vi "Aim test.vi"(0 "List box Aiming":string[](array[string]), 1 "Check path or camera":bool, 2 "Exposure":dbl, 5 "error in 3":errorcluster, 6 "Image":T1(plugin-control), 7 "Camera Refnum in":T3) -> (14 "Aiming Result":T2, 15 "Image 2":T1(plugin-control), 16 "Camera Refnum in 2":T3, 19 "error out 3":errorcluster)   [LabVIEW 2020]
uses:
  <vilib>/userdefined/High Color/IMAQdx.ctl
  <vilib>/vision/NI_Vision_Development_Module.lvlib
  <vilib>/vision/driver/NI_Vision_Acquisition_Software.lvlib
  <resource>/objmgr/imaqdx.rc
  General/Daq code/S-IO Channel List.ctl
panel:
  out "Elaphsed time":dbl
  out "millisecond timer value":u32
  out "Aiminjg name":string
  out "Y axis distance to move :":dbl
  out "X axis distance to move :":dbl
  out "RESULT":bool caption="Result"
  out "Y direction":bool
  out "X direction":bool
  out "Y":i64
  out "X":i64
  out "Y":i64
  out "X":i64
  in  "Boolean":bool
  out "Buffer Number":u32
  out "Frame Rate":dbl(knob) scale=0.0..100.0
  in  "Transperancy":dbl(slide) scale=0.0..1.0
  out "new picture":picture
  in  "stop":bool
  out "Cross Hair Coordinates 2":cluster{"X":i32, "Y":i32}
  out "Image Out 4":T1(plugin-control)
  out "Particle Measurements (Pixels) 4":dbl[][](array[numeric]) format="%.2f"
  out "Particle Measurements (Pixels) 3":dbl[][](array[numeric]) format="%.2f"
  out "Cross Hair Coordinates":cluster{"X":i32, "Y":i32}
  out "Particle Measurements (Pixels) 2":dbl[][](array[numeric]) format="%.2f"
  out "Particle Measurements (Pixels)":dbl[][](array[numeric]) format="%.2f"
  out "error out 2":errorcluster
  out "Image Out 3":T1(plugin-control)
  # "Status"
  # "Expected Value"
  # "Actual Value"
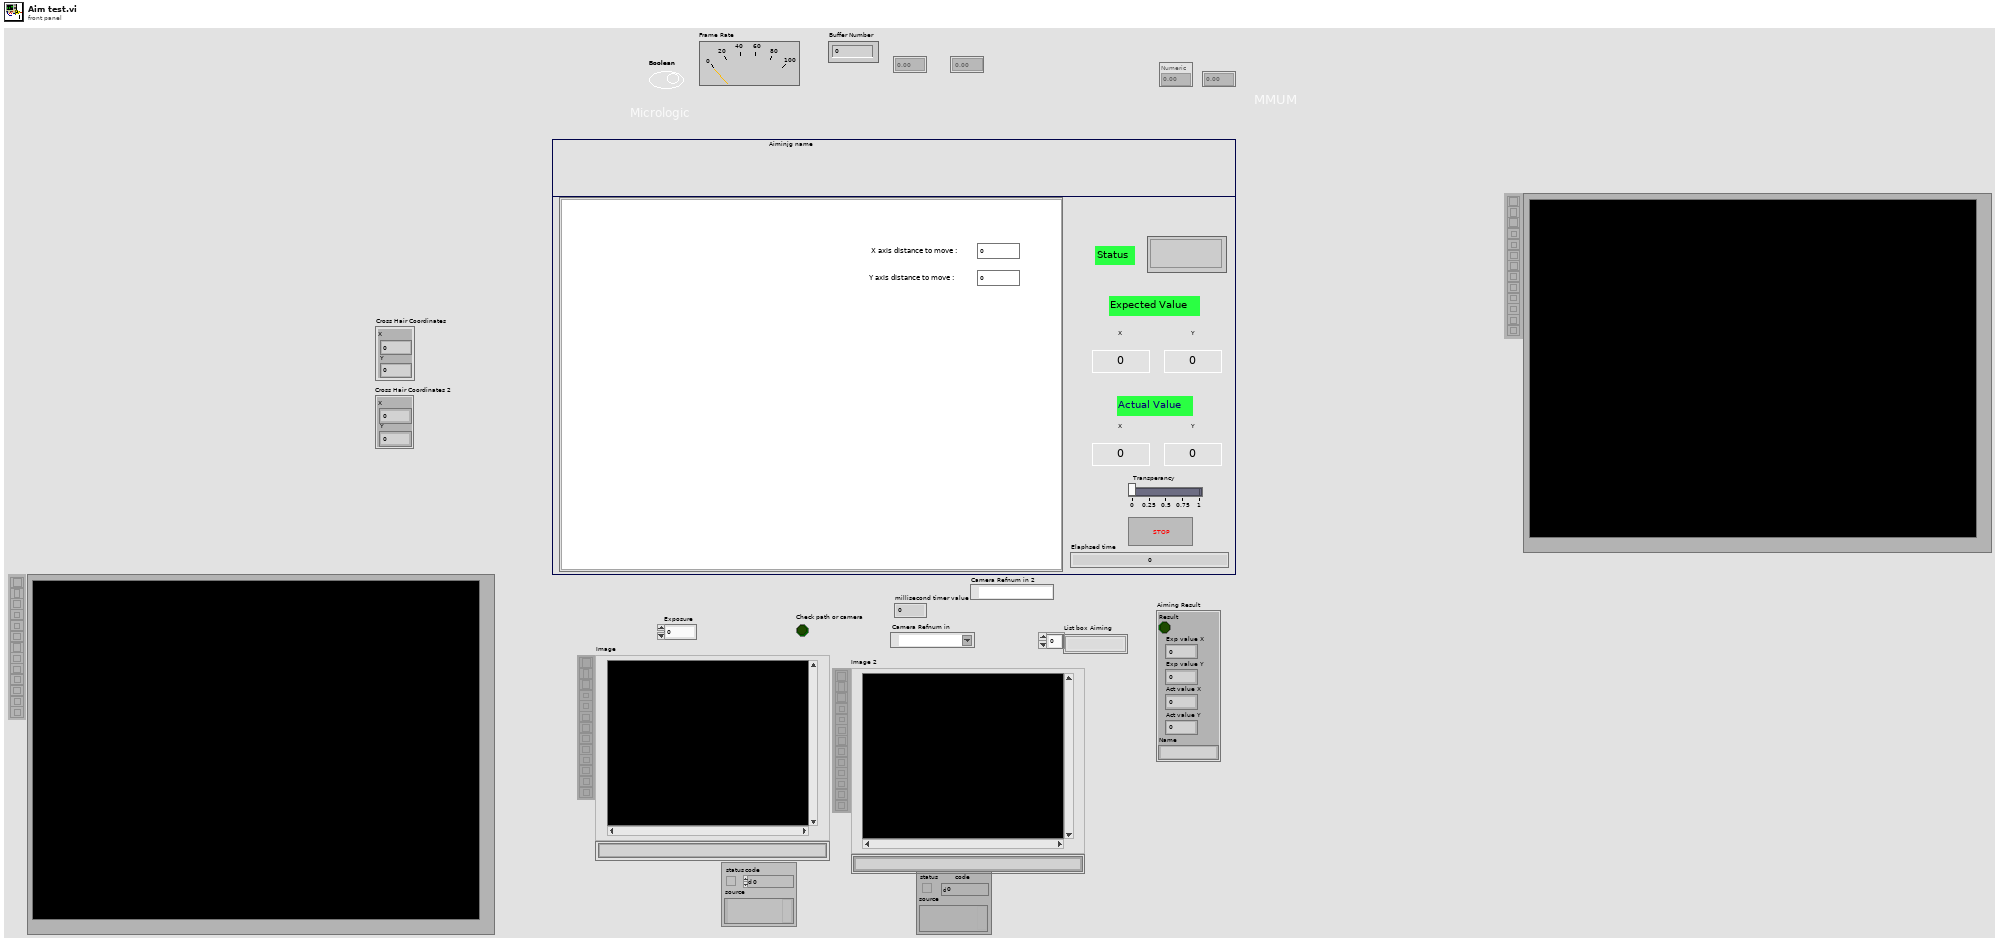
[diagram p1: front panel]
types:
  T1 = typedef "IMAQ Image.ctl" = refnum<image>
  T2 = cluster{"Result":bool, "Exp value X":i64, "Exp value Y":i64, "Act value X ":i64, "Act value Y ":i64, "Name":string}
  T3 = typedef "IMAQdx.ctl" = refnum<k21>
  T4 = typedef "Image Type" = u32
  T5 = typedef "Particle Parameters" = i32
  T6 = typedef "S-IO Channel List.ctl" = enum16{"Initialsation", "Reset All DOs", "Reset all expet lamp", "Read DI", "Read DI - line name", "Write DO", "Write DO - Line name", "Read DO", "Close"}
  T7 = cluster{"Left":i32, "Top":i32, "Right":i32, "Bottom":i32}
  T8 = typedef "imagedata.ctl" = cluster{"image type":i32, "image depth":i32, "image":u8[], "mask":u8[], "colors":u32[], "Rectangle":cluster{"left":i16, "top":i16, "right":i16, "bottom":i16}}
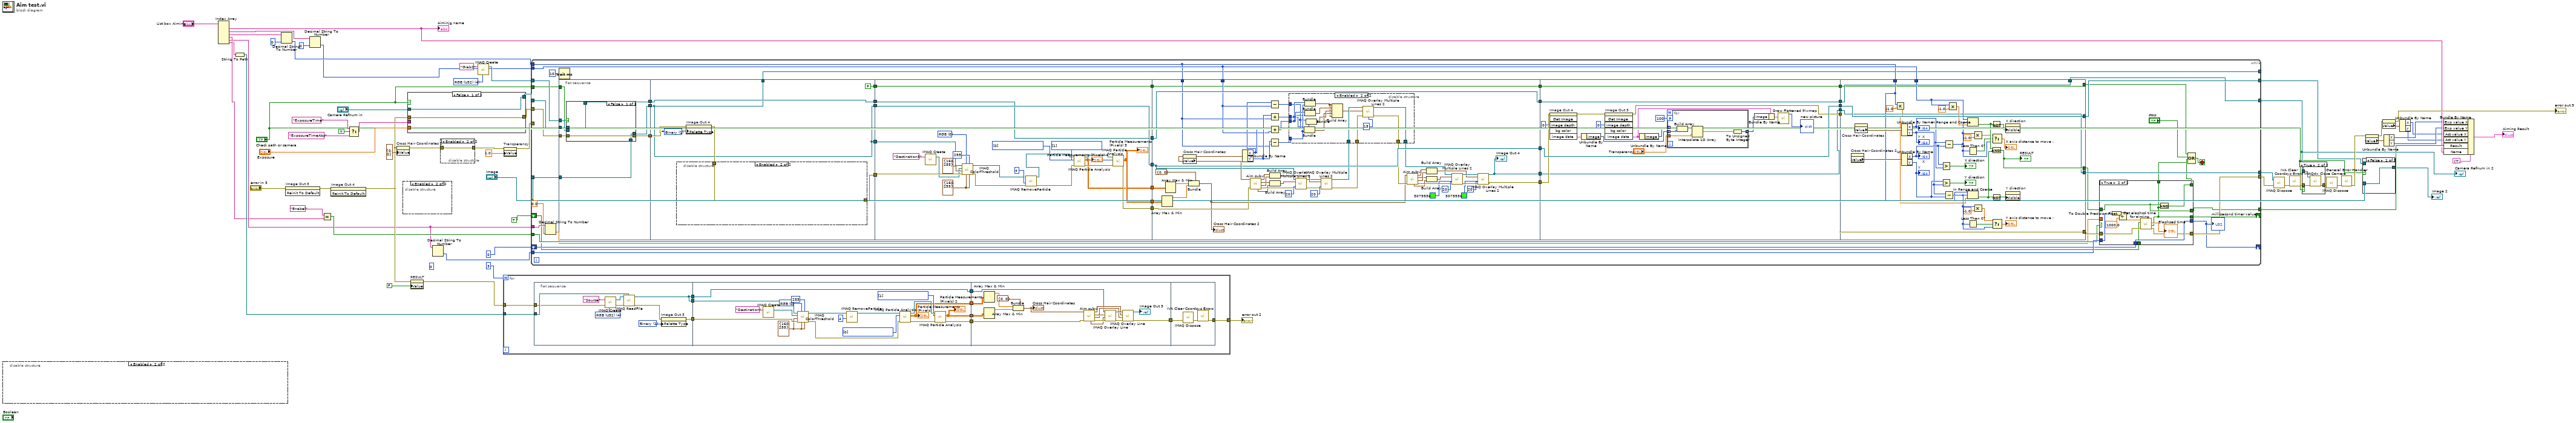
[diagram p0: block diagram]
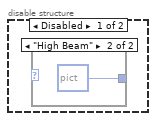
[diagram p3: hidden frame]
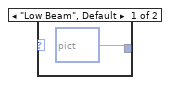
[diagram p4: hidden frame]
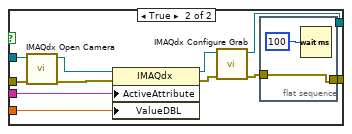
[diagram p6: hidden frame]
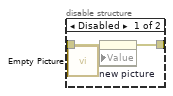
[diagram p7: hidden frame]
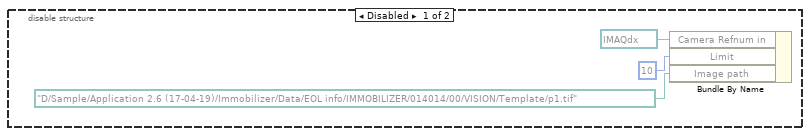
[diagram p8: hidden frame]
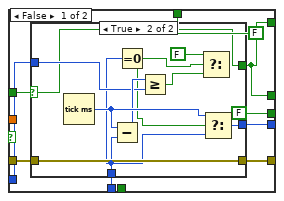
[diagram p9: hidden frame]
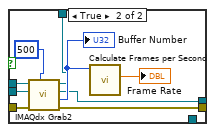
[diagram p11: hidden frame]
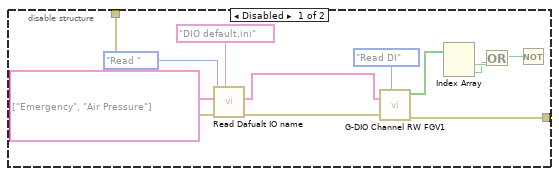
[diagram p12: hidden frame]
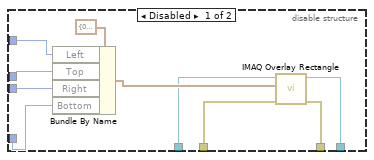
[diagram p13: hidden frame]
diagram:
  (unwired) i64 0 ("time out")
  w44 = T4 4 items=["Grayscale (U8)", "Grayscale (I16)", "Grayscale (SGL)", "Complex (CSG)", "RGB (U32)", "HSL (U32)", "RGB (U64)", "Grayscale (U16)"] ("Image Type")
  n1 = disable-structure shown="Enabled" {
    frame Disabled {
      n2 = Bundle By Name("Camera Refnum in"=T3 "cam1", "Limit"=i64 10, "Image path"=path "D:/Sample/Application 2.6 (17-04-19)/Immobilizer/Data/EOL info/IMMOBILIZER/014014/00/VISION/Template/p1.tif") -> ()  [unwired: 1 in, 1 out]
    }
    frame Enabled {
    }
  }
  n3 = Index Array(array="List box Aiming") -> (element #1=w20:string, element #2=w26:string, element #3=w27:string, element #4=w2:string, element #5=w3:string, element #6=w1:string)  [unwired: 6 in]
  "Aiminjg name" <- w20
  n4 = String To Path(string=w1) -> (path=w22:path)
  n5 = Decimal String To Number(string=w27, default (0L)=i64 0 ("Limit B")) -> (number=w25:i64)  [unwired: 1 in, 1 out]
  n6 = invoke on="Image Out 3" class="ImageControl" method="Reinit To Default"(error in="error in 3") -> (error out=w32:errorcluster)  [unwired: 2 in, 2 out]
  n7 = Decimal String To Number(string=w26, default (0L)=i64 0 ("Limit B")) -> (number=w24:i64)  [unwired: 1 in, 1 out]
  n8 = Equal?(x="Enabel" ("element"), y=w2) -> (x = y?=w4:bool)
  n9 = invoke on="Image Out 4" class="ImageControl" method="Reinit To Default"(error in=w32) -> (error out=w31:errorcluster)  [unwired: 2 in, 2 out]
  n10 = Select(t="ExposureTime" ("ActiveAttribute"), s=TRUE, f="ExposureTimeAbs" ("ActiveAttribute")) -> (s? t:f=w37:string)
  n11 = property on="Cross Hair Coordinates 2" class="Clust (strict)"(error in=w31, "Value"=cluster{"X":i32, "Y":i32} {"X"=0, "Y"=0} ("Cross Hair Coordinates 2")) -> (error out=w47:errorcluster)  [unwired: 1 in, 1 out]
  n12 = disable-structure shown="Enabled" {
    frame Disabled {
      n13 = case shown="\"High Beam\"" {
        selector: _ -> [_ _]
        tunnel: [picture bytes[1461630] ("new picture") picture bytes[1461630] ("new picture")] -> _
        frame "Low Beam", Default {
        }
        frame "High Beam" {
        }
      }
    }
    frame Enabled {
    }
  }
  n14 = case shown="False" "Check path or camera" {
    tunnel: [w70 w81] -> w63
    tunnel: "Camera Refnum in" -> [w70 w76]
    tunnel: [w69 w74] -> w43
    tunnel: w37 -> [_ w73]
    tunnel: w31 -> [w69 w72]
    tunnel: "Exposure" -> [_ w71]
    frame False {
    }
    frame True {
      n15 = call <vilib>:"IMAQdx Open Camera.vi"("error in"=w72, "Session In"=w76) -> ("error out"=w79:errorcluster, "Session Out"=w80:T3)  [unwired: 1 in, 7 out]
      n16 = property class="IMAQdx"(reference=w80, error in=w79, "ActiveAttribute"=w73, "ValueDBL"=w71) -> (reference out=w78:T3, error out=w77:errorcluster)
      n17 = call <vilib>:"IMAQdx Configure Grab.vi"("error in"=w77, "Session In"=w78) -> ("error out"=w75:errorcluster, "Session Out"=w81:T3)  [unwired: 1 in, 7 out]
      n18 = flat-sequence {
        tunnel: [w83] -> w74
        tunnel: w75 -> [w83]
        frame #0 {
          n19 = Wait (ms)(milliseconds to wait=u32 100) -> ()  [unwired: 1 out]
        }
      }
    }
  }
  n20 = property on="RESULT" class="Bool (strict)"(error in=w31, "Value"=FALSE ("RESULT")) -> (error out=w53:errorcluster)  [unwired: 1 in, 1 out]
  n21 = Decimal String To Number(string=w3) -> (number=w6:i32)  [unwired: 2 in, 1 out]
  n22 = disable-structure shown="Enabled" {
    disable-tunnel: w47 -> [w86 w87]
    disable-tunnel: [w85 w87] -> w46
    frame Disabled {
      n23 = call "Empty Picture"() -> ("empty picture"=w84:picture)
      n24 = property on="new picture" class="Pict"(error in=w86, "Value"=w84) -> (error out=w85:errorcluster)  [unwired: 1 in, 1 out]
    }
    frame Enabled {
    }
  }
  n25 = call "IMAQ Create"("Image Name"="Grab2", "Image Type"=w44) -> ("New Image"=w51:T1)  [unwired: 2 in, 2 out]
  n26 = for {
    N: 3 -> [_]
    tunnel: w22 -> [w90]
    tunnel: [w89] -> w49
    tunnel: w53 -> [w88]
    n27 = flat-sequence {
      tunnel: [w101] -> w98
      tunnel: [w103] -> w97
      tunnel: [w101] -> w96
      tunnel: w90 -> [w100]
      tunnel: w88 -> [w99]
      tunnel: w98 -> [w109]
      tunnel: w97 -> [w126]
      tunnel: [w119] -> w95
      tunnel: [w118] -> w94
      tunnel: [w117] -> w93
      tunnel: [w116] -> w92
      tunnel: w96 -> [w116]
      tunnel: w95 -> [w142]
      tunnel: [w130] -> w91
      tunnel: w94 -> [w134]
      tunnel: w93 -> [w133]
      tunnel: w92 -> [w132]
      tunnel: w91 -> [w147]
      tunnel: [w145] -> w89
      frame #0 {
        w105 = u32 1 items=["Grayscale", "Binary", "Gradient", "Rainbow", "Temperature", "User Defined", "Binary 16 Bit", "Gradient 16 Bit", "Rainbow 16 Bit", "Temperature 16 Bit", "User Defined 16 Bit"] ("Palette Type")
        w106 = T4 4 items=["Grayscale (U8)", "Grayscale (I16)", "Grayscale (SGL)", "Complex (CSG)", "RGB (U32)", "HSL (U32)", "RGB (U64)", "Grayscale (U16)"] ("Image Type")
        n28 = call "IMAQ Create"("Image Name"="Source", "Image Type"=w106, "error in (no error)"=w99) -> ("New Image"=w108:T1, "error out"=w107:errorcluster)  [unwired: 1 in, 1 out]
        n29 = call "IMAQ ReadFile"("File Path"=w100, "error in (no error)"=w107, "Image"=w108) -> ("error out"=w104:errorcluster, "Image Out"=w101:T1)  [unwired: 2 in, 5 out]
        n30 = property on="Image Out 3" class="ImageControl"(error in=w104, "Palette:Palette Type"=w105) -> (error out=w103:errorcluster)  [unwired: 1 in, 1 out]
      }
      frame #1 {
        w111 = u16 0 items=["RGB", "HSL", "HSV", "HSI"] ("Color Mode")
        w121 = T5[] [1] items=["Center of Mass X", "Center of Mass Y", "First Pixel X", "First Pixel Y", "Bounding Rect Left", "Bounding Rect Top", "Bounding Rect Right", "Bounding Rect Bottom", "Max Feret Diameter Start X", "Max Feret Diameter Start Y", "Max Feret Diameter End X", "Max Feret Diameter End Y", "Max Horiz. Segment Length Left", "Max Horiz. Segment Length Right", "Max Horiz. Segment Length Row", "-", "Bounding Rect Width", "Bounding Rect Height", "Bounding Rect Diagonal", "Perimeter", "Convex Hull Perimeter", "Holes' Perimeter", "Max Feret Diameter", "Equivalent Ellipse Major Axis", "Equivalent Ellipse Minor Axis", "Equivalent Ellipse Minor Axis (Feret)", "Equivalent Rect Long Side", "Equivalent Rect Short Side", "Equivalent Rect Diagonal", "Equivalent Rect Short Side (Feret)", "Average Horiz. Segment Length", "Average Vert. Segment Length", "Hydraulic Radius", "Waddel Disk Diameter", "-", "Area", "Holes' Area", "Particle & Holes' Area", "Convex Hull Area", "Image Area", "-", "Number of Holes", "Number of Horiz. Segments", "Number of Vert. Segments", "-", "Orientation", "Max Feret Diameter Orientation", "-", "% Area/Image Area", "% Area/(Particle & Holes' Area)", "Ratio of Equivalent Ellipse Axes", "Ratio of Equivalent Rect Sides", "-", "Elongation Factor", "Compactness Factor", "Heywood Circularity Factor", "Type Factor", "-", "Sum X", "Sum Y", "Sum XX", "Sum XY", "Sum YY", "Sum XXX", "Sum XXY", "Sum XYY", "Sum YYY", "-", "Moment of Inertia XX", "Moment of Inertia XY", "Moment of Inertia YY", "Moment of Inertia XXX", "Moment of Inertia XXY", "Moment of Inertia XYY", "Moment of Inertia YYY", "Norm. Moment of Inertia XX", "Norm. Moment of Inertia XY", "Norm. Moment of Inertia YY", "Norm. Moment of Inertia XXX", "Norm. Moment of Inertia XXY", "Norm. Moment of Inertia XYY", "Norm. Moment of Inertia YYY", "Hu Moment 1", "Hu Moment 2", "Hu Moment 3", "Hu Moment 4", "Hu Moment 5", "Hu Moment 6", "Hu Moment 7"] ("Pixel Measurements")
        w113 = cluster{"Lower value":i32, "Upper value":i32} {"Lower value"=160, "Upper value"=255} ("Red or Hue Range")
        w127 = T5[] [0] items=["Center of Mass X", "Center of Mass Y", "First Pixel X", "First Pixel Y", "Bounding Rect Left", "Bounding Rect Top", "Bounding Rect Right", "Bounding Rect Bottom", "Max Feret Diameter Start X", "Max Feret Diameter Start Y", "Max Feret Diameter End X", "Max Feret Diameter End Y", "Max Horiz. Segment Length Left", "Max Horiz. Segment Length Right", "Max Horiz. Segment Length Row", "-", "Bounding Rect Width", "Bounding Rect Height", "Bounding Rect Diagonal", "Perimeter", "Convex Hull Perimeter", "Holes' Perimeter", "Max Feret Diameter", "Equivalent Ellipse Major Axis", "Equivalent Ellipse Minor Axis", "Equivalent Ellipse Minor Axis (Feret)", "Equivalent Rect Long Side", "Equivalent Rect Short Side", "Equivalent Rect Diagonal", "Equivalent Rect Short Side (Feret)", "Average Horiz. Segment Length", "Average Vert. Segment Length", "Hydraulic Radius", "Waddel Disk Diameter", "-", "Area", "Holes' Area", "Particle & Holes' Area", "Convex Hull Area", "Image Area", "-", "Number of Holes", "Number of Horiz. Segments", "Number of Vert. Segments", "-", "Orientation", "Max Feret Diameter Orientation", "-", "% Area/Image Area", "% Area/(Particle & Holes' Area)", "Ratio of Equivalent Ellipse Axes", "Ratio of Equivalent Rect Sides", "-", "Elongation Factor", "Compactness Factor", "Heywood Circularity Factor", "Type Factor", "-", "Sum X", "Sum Y", "Sum XX", "Sum XY", "Sum YY", "Sum XXX", "Sum XXY", "Sum XYY", "Sum YYY", "-", "Moment of Inertia XX", "Moment of Inertia XY", "Moment of Inertia YY", "Moment of Inertia XXX", "Moment of Inertia XXY", "Moment of Inertia XYY", "Moment of Inertia YYY", "Norm. Moment of Inertia XX", "Norm. Moment of Inertia XY", "Norm. Moment of Inertia YY", "Norm. Moment of Inertia XXX", "Norm. Moment of Inertia XXY", "Norm. Moment of Inertia XYY", "Norm. Moment of Inertia YYY", "Hu Moment 1", "Hu Moment 2", "Hu Moment 3", "Hu Moment 4", "Hu Moment 5", "Hu Moment 6", "Hu Moment 7"] ("Pixel Measurements")
        n31 = call "IMAQ Create"("Image Name"="Destination") -> ("New Image"=w123:T1)  [unwired: 3 in, 2 out]
        n32 = call "IMAQ ColorThreshold"("Blue or Luma or Val or Inten Range"=w113, "Replace Value"=255, "Green or Sat Range"=w113, "Color Mode"=w111, "error in (no error)"=w126, "Red or Hue Range"=w113, "Image Dst"=w123, "Image Src"=w109) -> ("error out"=w125:errorcluster, "Image Dst Out"=w110:T1)  [unwired: 2 in]
        n33 = call "IMAQ RemoveParticle"("Number of Erosion"=4, "Image Src"=w110) -> ("Image Dst Out"=w115:T1)  [unwired: 5 in, 4 out]
        n34 = call "IMAQ Particle Analysis"("error in (no error)"=w125, "Pixel Measurements"=w127, "Image"=w115) -> ("error out"=w120:errorcluster, "Particle Measurements (Pixels)"=w118:dbl[][], "Image Out (duplicate)"=w122:T1)  [unwired: 3 in, 3 out]
        "Particle Measurements (Pixels)" <- w118
        n35 = call "IMAQ Particle Analysis"("error in (no error)"=w120, "Pixel Measurements"=w121, "Image"=w122) -> ("error out"=w119:errorcluster, "Particle Measurements (Pixels)"=w117:dbl[][])  [unwired: 3 in, 4 out]
        "Particle Measurements (Pixels) 2" <- w117
      }
      frame #2 {
        n36 = Array Max & Min(array=w134) -> (max value=w144:dbl)  [unwired: 3 out]
        n37 = Array Max & Min(array=w133) -> (max value=w143:dbl)  [unwired: 3 out]
        n38 = Bundle(cluster=cluster{"X":i32, "Y":i32} {"X"=0, "Y"=0} ("Cross Hair Coordinates 2"), "X"=w144, "Y"=w143) -> (w128:cluster{"X":i32, "Y":i32})
        "Cross Hair Coordinates" <- w128
        n39 = call "Aim subvi.vi"("Coordinates"=w128, "error in (no error)"=w142) -> ("Cluster 3"=w135:cluster{"X":i32, "Y":i32}, "Cluster 2"=w138:cluster{"X":i32, "Y":i32}, "Cluster 4"=w137:cluster{"X":i32, "Y":i32}, "Cluster"=w136:cluster{"X":i32, "Y":i32}, "error out"=w141:errorcluster)  [unwired: 4 in]
        n40 = call "IMAQ Overlay Line"("error in (no error)"=w141, "End Point"=w135, "Start Point"=w137, "Image"=w132) -> ("error out"=w140:errorcluster, "Image Out"=w139:T1)  [unwired: 6 in]
        n41 = call "IMAQ Overlay Line"("error in (no error)"=w140, "End Point"=w136, "Start Point"=w138, "Image"=w139) -> ("error out"=w130:errorcluster, "Image Out"=→"Image Out 3":T1)  [unwired: 6 in]
      }
      frame #3 {
        n42 = call "IMAQ Dispose"("error in (no error)"=w147) -> ("error out"=w146:errorcluster)  [unwired: 2 in, 3 out]
        n43 = call <vilib>:"IVA Clear Coordsys Errors.vi"("error in (no error)"=w146) -> ("error out"=w145:errorcluster)  [unwired: 10 in]
      }
    }
  }
  "error out 2" <- w49
  n44 = property on="Transperancy" class="Slide (strict)"(error in=w46, "Value"=1.0 ("Transperancy")) -> (error out=w57:errorcluster)  [unwired: 1 in, 1 out]
  n45 = while {
    tunnel: w43 -> [w191]
    tunnel: [w170] -> w59
    tunnel: w24 -> [w172]
    tunnel: w57 -> [_]
    tunnel: [w173] -> w50
    tunnel: w25 -> [w171]
    shift-right: [w168] -> _
    shift-left: u32 0 ("millisecond timer value") -> [w161]
    tunnel: w6 -> [w167]
    tunnel: w63 -> [w190]
    tunnel: [w178] -> w41
    tunnel: w51 -> [w177]
    tunnel: [w185] -> w10
    tunnel: w3 -> [w160]
    tunnel: w4 -> [w158]
    shift-right: [w157] -> _
    shift-left: TRUE ("Elaphshed time") -> [w156]
    tunnel: [w152] -> w35
    tunnel: "Check path or camera" -> [w150]
    tunnel: "Image" -> [w149]
    tunnel: [w148] -> _
    stop <- w180 stop-if-true
    n46 = Decimal String To Number(string=w160, default (0L)=0.0) -> (number=w155:dbl)  [unwired: 1 in, 1 out]
    n47 = flat-sequence {
      tunnel: [w239] -> w193
      tunnel: [w238] -> w192
      tunnel: w191 -> [w243]
      tunnel: w190 -> [w242]
      tunnel: [w241] -> w186
      tunnel: w177 -> [w240]
      tunnel: w150 -> [w237]
      tunnel: w149 -> [w236]
      tunnel: [w256] -> w201
      tunnel: [w259] -> w200
      tunnel: [w256] -> w199
      tunnel: w193 -> [w256]
      tunnel: w192 -> [w262]
      tunnel: [w261] -> w187
      tunnel: w186 -> [w261]
      tunnel: [FALSE] -> w163
      tunnel: [w256] -> w148
      tunnel: w201 -> [w276]
      tunnel: w200 -> [w285]
      tunnel: [w293] -> w198
      tunnel: [w288] -> w197
      tunnel: [w289] -> w196
      tunnel: [w292] -> w195
      tunnel: w199 -> [w292]
      tunnel: [w287] -> w188
      tunnel: w187 -> [w287]
      tunnel: [w280] -> w164
      tunnel: w163 -> [w280]
      tunnel: w198 -> [w331]
      tunnel: w197 -> [w345]
      tunnel: w196 -> [w344]
      tunnel: w195 -> [w332]
      tunnel: [w343] -> w189
      tunnel: w188 -> [w343]
      tunnel: [w332] -> w184
      tunnel: [w305] -> w176
      tunnel: [w307] -> w175
      tunnel: w172 -> [w333]
      tunnel: w171 -> [w301]
      tunnel: [w299] -> w165
      tunnel: w164 -> [w299]
      tunnel: w189 -> [w378]
      tunnel: w184 -> [w377]
      tunnel: [w378] -> w183
      tunnel: [w377] -> w182
      tunnel: [w376] -> w181
      tunnel: w176 -> [w375]
      tunnel: w175 -> [w374]
      tunnel: [w374] -> w174
      tunnel: [w373] -> w166
      tunnel: w165 -> [w373]
      tunnel: [w427] -> w169
      tunnel: [w428] -> w185
      tunnel: [w429] -> w178
      tunnel: w183 -> [w429]
      tunnel: w182 -> [w428]
      tunnel: w181 -> [w427]
      tunnel: w172 -> [w402]
      tunnel: [w401] -> w153
      tunnel: w174 -> [w400]
      tunnel: [w400] -> w173
      tunnel: w171 -> [w398]
      tunnel: [w396] -> w162
      tunnel: w166 -> [w396]
      frame #0 {
        n48 = case shown="False" w237 {
          tunnel: w243 -> [w245 w253]
          tunnel: w242 -> [w246 w252]
          tunnel: [w246 w251] -> w241
          tunnel: w240 -> [_ w250]
          tunnel: [w244 w248] -> w239
          tunnel: [w245 w247] -> w238
          tunnel: w236 -> [w244 _]
          frame False {
          }
          frame True {
            n49 = call <vilib>:"IMAQdx Grab2.vi"("Timeout (ms)"=500, "error in"=w253, "Image In"=w250, "Session In"=w252) -> ("error out"=w247:errorcluster, "Buffer Number Out"=w254:u32, "Image Out"=w248:T1, "Session Out"=w251:T3)  [unwired: 4 in]
            "Buffer Number" <- w254
            n50 = call <vilib>:"Calculate Frames per Second.vi"("Buffer Number"=w254) -> ("Processed Frames/s"=→"Frame Rate":dbl)  [unwired: 8 in, 2 out]
          }
        }
      }
      frame #1 {
        w257 = u32 1 items=["Grayscale", "Binary", "Gradient", "Rainbow", "Temperature", "User Defined", "Binary 16 Bit", "Gradient 16 Bit", "Rainbow 16 Bit", "Temperature 16 Bit", "User Defined 16 Bit"] ("Palette Type")
        n51 = property on="Image Out 4" class="ImageControl"(error in=w262, "Palette:Palette Type"=w257) -> (error out=w260:errorcluster)  [unwired: 1 in, 1 out]
        n52 = disable-structure shown="Enabled" {
          disable-tunnel: w260 -> [w270 w275]
          disable-tunnel: [w269 w275] -> w259
          frame Disabled {
            n53 = call "Read Dafualt IO name.vi"("Default Control"="DIO default.ini", "error in (no error)"=w270, "Input/output name"=string[] ["Emergency", "Air Pressure"], "Read/ Write"=enum16{"INI", "Read ", "Write"}."Read ") -> ("error out"=w263:errorcluster, "Value"=w274:string[])  [unwired: 6 in]
            n54 = call "G-DIO Channel RW FGV1.vi"("Command"=S-IO_Channel_List."Read DI", "error in (no error)"=w263, "DIO Names"=w274) -> ("error out"=w269:errorcluster, "Write status"=w267:bool[])  [unwired: 6 in, 1 out]
            n55 = Index Array(array=w267) -> (element #1=w266:bool, element #2=w265:bool)  [unwired: 2 in]
            n56 = Or(x=w266, y=w265) -> (x .or. y?=w264:bool)
            n57 = Not(x=w264) -> ()  [unwired: 1 out]
          }
          frame Enabled {
          }
        }
      }
      frame #2 {
        w279 = u16 0 items=["RGB", "HSL", "HSV", "HSI"] ("Color Mode")
        w295 = T5[] [1] items=["Center of Mass X", "Center of Mass Y", "First Pixel X", "First Pixel Y", "Bounding Rect Left", "Bounding Rect Top", "Bounding Rect Right", "Bounding Rect Bottom", "Max Feret Diameter Start X", "Max Feret Diameter Start Y", "Max Feret Diameter End X", "Max Feret Diameter End Y", "Max Horiz. Segment Length Left", "Max Horiz. Segment Length Right", "Max Horiz. Segment Length Row", "-", "Bounding Rect Width", "Bounding Rect Height", "Bounding Rect Diagonal", "Perimeter", "Convex Hull Perimeter", "Holes' Perimeter", "Max Feret Diameter", "Equivalent Ellipse Major Axis", "Equivalent Ellipse Minor Axis", "Equivalent Ellipse Minor Axis (Feret)", "Equivalent Rect Long Side", "Equivalent Rect Short Side", "Equivalent Rect Diagonal", "Equivalent Rect Short Side (Feret)", "Average Horiz. Segment Length", "Average Vert. Segment Length", "Hydraulic Radius", "Waddel Disk Diameter", "-", "Area", "Holes' Area", "Particle & Holes' Area", "Convex Hull Area", "Image Area", "-", "Number of Holes", "Number of Horiz. Segments", "Number of Vert. Segments", "-", "Orientation", "Max Feret Diameter Orientation", "-", "% Area/Image Area", "% Area/(Particle & Holes' Area)", "Ratio of Equivalent Ellipse Axes", "Ratio of Equivalent Rect Sides", "-", "Elongation Factor", "Compactness Factor", "Heywood Circularity Factor", "Type Factor", "-", "Sum X", "Sum Y", "Sum XX", "Sum XY", "Sum YY", "Sum XXX", "Sum XXY", "Sum XYY", "Sum YYY", "-", "Moment of Inertia XX", "Moment of Inertia XY", "Moment of Inertia YY", "Moment of Inertia XXX", "Moment of Inertia XXY", "Moment of Inertia XYY", "Moment of Inertia YYY", "Norm. Moment of Inertia XX", "Norm. Moment of Inertia XY", "Norm. Moment of Inertia YY", "Norm. Moment of Inertia XXX", "Norm. Moment of Inertia XXY", "Norm. Moment of Inertia XYY", "Norm. Moment of Inertia YYY", "Hu Moment 1", "Hu Moment 2", "Hu Moment 3", "Hu Moment 4", "Hu Moment 5", "Hu Moment 6", "Hu Moment 7"] ("Pixel Measurements")
        w282 = cluster{"Lower value":i32, "Upper value":i32} {"Lower value"=160, "Upper value"=255} ("Red or Hue Range")
        w298 = T5[] [0] items=["Center of Mass X", "Center of Mass Y", "First Pixel X", "First Pixel Y", "Bounding Rect Left", "Bounding Rect Top", "Bounding Rect Right", "Bounding Rect Bottom", "Max Feret Diameter Start X", "Max Feret Diameter Start Y", "Max Feret Diameter End X", "Max Feret Diameter End Y", "Max Horiz. Segment Length Left", "Max Horiz. Segment Length Right", "Max Horiz. Segment Length Row", "-", "Bounding Rect Width", "Bounding Rect Height", "Bounding Rect Diagonal", "Perimeter", "Convex Hull Perimeter", "Holes' Perimeter", "Max Feret Diameter", "Equivalent Ellipse Major Axis", "Equivalent Ellipse Minor Axis", "Equivalent Ellipse Minor Axis (Feret)", "Equivalent Rect Long Side", "Equivalent Rect Short Side", "Equivalent Rect Diagonal", "Equivalent Rect Short Side (Feret)", "Average Horiz. Segment Length", "Average Vert. Segment Length", "Hydraulic Radius", "Waddel Disk Diameter", "-", "Area", "Holes' Area", "Particle & Holes' Area", "Convex Hull Area", "Image Area", "-", "Number of Holes", "Number of Horiz. Segments", "Number of Vert. Segments", "-", "Orientation", "Max Feret Diameter Orientation", "-", "% Area/Image Area", "% Area/(Particle & Holes' Area)", "Ratio of Equivalent Ellipse Axes", "Ratio of Equivalent Rect Sides", "-", "Elongation Factor", "Compactness Factor", "Heywood Circularity Factor", "Type Factor", "-", "Sum X", "Sum Y", "Sum XX", "Sum XY", "Sum YY", "Sum XXX", "Sum XXY", "Sum XYY", "Sum YYY", "-", "Moment of Inertia XX", "Moment of Inertia XY", "Moment of Inertia YY", "Moment of Inertia XXX", "Moment of Inertia XXY", "Moment of Inertia XYY", "Moment of Inertia YYY", "Norm. Moment of Inertia XX", "Norm. Moment of Inertia XY", "Norm. Moment of Inertia YY", "Norm. Moment of Inertia XXX", "Norm. Moment of Inertia XXY", "Norm. Moment of Inertia XYY", "Norm. Moment of Inertia YYY", "Hu Moment 1", "Hu Moment 2", "Hu Moment 3", "Hu Moment 4", "Hu Moment 5", "Hu Moment 6", "Hu Moment 7"] ("Pixel Measurements")
        n58 = call "IMAQ Create"("Image Name"="Destination5") -> ("New Image"=w278:T1)  [unwired: 3 in, 2 out]
        n59 = call "IMAQ ColorThreshold"("Blue or Luma or Val or Inten Range"=w282, "Replace Value"=255, "Green or Sat Range"=w282, "Color Mode"=w279, "error in (no error)"=w285, "Red or Hue Range"=cluster{"Lower value":i32, "Upper value":i32} {"Lower value"=160, "Upper value"=255}, "Image Dst"=w278, "Image Src"=w276) -> ("error out"=w284:errorcluster, "Image Dst Out"=w277:T1)  [unwired: 2 in]
        n60 = call "IMAQ RemoveParticle"("error in (no error)"=w284, "Number of Erosion"=4, "Image Src"=w277) -> ("error out"=w286:errorcluster, "Image Dst Out"=w291:T1)  [unwired: 4 in, 3 out]
        n61 = call "IMAQ Particle Analysis"("error in (no error)"=w286, "Pixel Measurements"=w298, "Image"=w291) -> ("error out"=w294:errorcluster, "Particle Measurements (Pixels)"=w288:dbl[][], "Image Out (duplicate)"=w296:T1)  [unwired: 3 in, 3 out]
        "Particle Measurements (Pixels) 4" <- w288
        n62 = call "IMAQ Particle Analysis"("error in (no error)"=w294, "Pixel Measurements"=w295, "Image"=w296) -> ("error out"=w293:errorcluster, "Particle Measurements (Pixels)"=w289:dbl[][])  [unwired: 3 in, 4 out]
        "Particle Measurements (Pixels) 3" <- w289
      }
      frame #3 {
        n63 = Array Max & Min(array=w344) -> (max value=w346:dbl)  [unwired: 3 out]
        n64 = Array Max & Min(array=w345) -> (max value=w347:dbl)  [unwired: 3 out]
        n65 = property on="Cross Hair Coordinates" class="Clust (strict)"() -> ("Value"=w334:cluster{"X":i32, "Y":i32})  [unwired: 2 in, 2 out]
        n66 = Bundle(cluster=cluster{"X":i32, "Y":i32} {"X"=0, "Y"=0} ("Cross Hair Coordinates 2"), "X"=w347, "Y"=w346) -> (w300:cluster{"X":i32, "Y":i32})
        "Cross Hair Coordinates 2" <- w300
        n67 = Unbundle By Name(w334) -> ("X"=w339:i32, "Y"=w338:i32)
        n68 = call "Aim subvi.vi"("Coordinates"=w334, "error in (no error)"=w331) -> ("Cluster 3"=w329:cluster{"X":i32, "Y":i32}, "Cluster 2"=w322:cluster{"X":i32, "Y":i32}, "Cluster 4"=w330:cluster{"X":i32, "Y":i32}, "Cluster"=w321:cluster{"X":i32, "Y":i32}, "error out"=w335:errorcluster)  [unwired: 4 in]
        n69 = Subtract(x=w339, y=w333) -> (x-y=w340:i64)
        n70 = Add(x=w338, y=w301) -> (x+y=w337:i64)
        n71 = Add(x=w339, y=w333) -> (x+y=w341:i64)
        n72 = Subtract(x=w338, y=w301) -> (x-y=w336:i64)
        n73 = Build Array(w322, w321) -> (w325:cluster{"X":i32, "Y":i32}[])
        n74 = Build Array(w330, w329) -> (w328:cluster{"X":i32, "Y":i32}[])
        n75 = call "IMAQ Overlay Multiple Lines 2"("Image"=w332, "Line End Points"=w328, "error in (no error)"=w335, "Width"=u32 20) -> ("Image Out"=w320:T1, "error out"=w319:errorcluster)  [unwired: 10 in]
        n76 = call "IMAQ Overlay Multiple Lines 2"("Image"=w320, "Line End Points"=w325, "error in (no error)"=w319, "Width"=u32 20) -> ("Image Out"=w324:T1, "error out"=w323:errorcluster)  [unwired: 10 in]
        n77 = disable-structure shown="Enabled" {
          disable-tunnel: w341 -> [w355 w367]
          disable-tunnel: w340 -> [w354 w366]
          disable-tunnel: w337 -> [w353 w358]
          disable-tunnel: w336 -> [w352 w365]
          disable-tunnel: w324 -> [w351 w369]
          disable-tunnel: w323 -> [w350 w368]
          disable-tunnel: [w349 w371] -> w308
          disable-tunnel: [w348 w370] -> w306
          frame Disabled {
            n78 = Bundle By Name(cluster=T7 {"Left"=0, "Top"=0, "Right"=0, "Bottom"=0} ("Rectangle"), "Left"=w354, "Top"=w353, "Right"=w355, "Bottom"=w352) -> (w356:T7)
            n79 = call "IMAQ Overlay Rectangle"("error in (no error)"=w350, "Rectangle"=w356, "Image"=w351) -> ("error out"=w348:errorcluster, "Image Out"=w349:T1)  [unwired: 7 in]
          }
          frame Enabled {
            n80 = Bundle(w366, w365) -> (w362:cluster{i64, i64})  [unwired: 1 in]
            n81 = Bundle(w367, w365) -> (w361:cluster{i64, i64})  [unwired: 1 in]
            n82 = Bundle(w367, w358) -> (w364:cluster{i64, i64})  [unwired: 1 in]
            n83 = Bundle(w366, w358) -> (w363:cluster{i64, i64})  [unwired: 1 in]
            n84 = Build Array(w361, w364, w363, w362, w361) -> (w360:cluster{i64, i64}[])
            n85 = call "IMAQ Overlay Multiple Lines 2"("Image"=w369, "Line End Points"=w360, "error in (no error)"=w368, "Width"=u32 15) -> ("Image Out"=w371:T1, "error out"=w370:errorcluster)  [unwired: 10 in]
          }
        }
        n86 = call "Aim subvi.vi"("Coordinates"=w300, "error in (no error)"=w306) -> ("Cluster 3"=w302:cluster{"X":i32, "Y":i32}, "Cluster 2"=w315:cluster{"X":i32, "Y":i32}, "Cluster 4"=w310:cluster{"X":i32, "Y":i32}, "Cluster"=w316:cluster{"X":i32, "Y":i32}, "error out"=w309:errorcluster)  [unwired: 4 in]
        n87 = Build Array(w315, w316) -> (w314:cluster{"X":i32, "Y":i32}[])
        n88 = Build Array(w310, w302) -> (w311:cluster{"X":i32, "Y":i32}[])
        n89 = call "IMAQ Overlay Multiple Lines 2"("Image"=w308, "Line End Points"=w311, "Color"=u32 3079936, "error in (no error)"=w309, "Width"=u32 20) -> ("Image Out"=w317:T1, "error out"=w318:errorcluster)  [unwired: 9 in]
        n90 = call "IMAQ Overlay Multiple Lines 2"("Image"=w317, "Line End Points"=w314, "Color"=u32 3079936, "error in (no error)"=w318, "Width"=u32 20) -> ("Image Out"=w307:T1, "error out"=w305:errorcluster)  [unwired: 9 in]
        "Image Out 4" <- w307
      }
      frame #4 {
        n91 = invoke on="Image Out 4" class="ImageControl" method="Get Image"(error in=w375, "image depth"=0 ("Image Depth")) -> (error out=w389:errorcluster, "image data"=w388:T8)  [unwired: 4 in, 4 out]
        n92 = Unbundle By Name(w388) -> ("image"=w384:u8[])
        n93 = invoke on="Image Out 3" class="ImageControl" method="Get Image"(error in=w389, "image depth"=0 ("Image Depth")) -> (error out=w376:errorcluster, "image data"=w387:T8)  [unwired: 4 in, 4 out]
        n94 = Unbundle By Name(w387) -> ("image"=w383:u8[])
        n95 = for {
          tunnel: w384 -> [w395] mode=indexing
          tunnel: w383 -> [w394] mode=indexing
          tunnel: [w391] -> w382 mode=indexing
          tunnel: "Transperancy" -> [w390]
          workers-P: 100 -> [_]
          n96 = Build Array(w394, w395) -> (w393:u8[])
          n97 = Interpolate 1D Array(1:w390, 2:w393) -> (0:w392:dbl)
          n98 = To Unsigned Byte Integer(number=w392) -> (unsigned 8bit integer=w391:u8)
        }
        n99 = Bundle By Name(cluster=w387, "image"=w382) -> (w386:T8)
        n100 = call <vilib>:"Draw Flattened Pixmap.vi"("image data"=w386) -> ("new picture"=→"new picture":picture)  [unwired: 1 in, 7 out]
      }
      frame #5 {
        n101 = property on="Cross Hair Coordinates 2" class="Clust (strict)"() -> ("Value"=w403:cluster{"X":i32, "Y":i32})  [unwired: 2 in, 2 out]
        n102 = property on="Cross Hair Coordinates" class="Clust (strict)"() -> ("Value"=w407:cluster{"X":i32, "Y":i32})  [unwired: 2 in, 2 out]
        n103 = Multiply(x=w398, y=-1.0 ("upper limit")) -> (x*y=w397:dbl)
        n104 = Unbundle By Name(w407) -> ("X"=w409:i32, "Y"=w411:i32)
        "X" <- w409
        "Y" <- w411
        n105 = Unbundle By Name(w403) -> ("X"=w414:i32, "Y"=w413:i32)
        "Y" <- w413
        "X" <- w414
        n106 = Greater?(x=w414, y=w409) -> (0:→"X direction":bool)
        n107 = Greater?(x=w413, y=w411) -> (0:→"Y direction":bool)
        n108 = Subtract(x=w409, y=w414) -> (x-y=w422:i32)
        n109 = Subtract(x=w411, y=w413) -> (x-y=w420:i32)
        n110 = Multiply(x=w402, y=-1.0 ("upper limit")) -> (x*y=w408:dbl)
        n111 = In Range and Coerce(upper limit=w402, x=w422, lower limit=w408) -> (In Range?=w423:bool)  [unwired: 1 out]
        n112 = In Range and Coerce(upper limit=w398, x=w420, lower limit=w397) -> (In Range?=w424:bool)  [unwired: 1 out]
        n113 = Less Than 0?(x=w422) -> (x < 0?=w415:bool)
        n114 = Less Than 0?(x=w420) -> (x < 0?=w419:bool)
        n115 = Multiply(x=w422, y=-1.0 ("upper limit")) -> (x*y=w417:dbl)
        n116 = Multiply(x=w420, y=-1.0 ("upper limit")) -> (x*y=w418:dbl)
        n117 = Not(x=w423) -> (.not. x?=w425:bool)
        n118 = And(x=w423, y=w424) -> (x .and. y?=w401:bool)
        "RESULT" <- w401
        n119 = Not(x=w424) -> (.not. x?=w426:bool)
        n120 = Select(t=w417, s=w415, f=w422) -> (s? t:f=→"X axis distance to move :":dbl)
        n121 = Select(t=w418, s=w419, f=w420) -> (s? t:f=→"Y axis distance to move :":dbl)
        n122 = property on="X direction" class="Bool"("Visible"=w425) -> ()  [unwired: 2 in, 2 out]
        n123 = property on="Y direction" class="Bool"("Visible"=w426) -> ()  [unwired: 2 in, 2 out]
      }
    }
    n124 = Wait (ms)(milliseconds to wait=u32 10) -> ()  [unwired: 1 out]
    n125 = case shown="True" w158 {
      tunnel: [w210 w233] -> w170
      tunnel: w169 -> [w209 w234]
      tunnel: [w208 w235] -> w168
      tunnel: w167 -> [w207 w229]
      tunnel: w153 -> [w206 w230]
      tunnel: w161 -> [w205 w235]
      tunnel: [w203 w231] -> w154
      tunnel: [FALSE ("Elaphshed time") w226] -> w157
      tunnel: w156 -> [_ w232]
      tunnel: w155 -> [_ _]
      tunnel: [w203 w230] -> w152
      tunnel: [FALSE ("Elaphshed time") w226] -> w151
      frame False {
        n126 = case shown="True" w206 {
          selector: w206 -> [w212 w214]
          tunnel: [w213 w223] -> w210
          tunnel: w209 -> [w213 w223]
          tunnel: [w212 w214] -> w203
          tunnel: [w211 w220] -> w208
          tunnel: w205 -> [w211 w216]
          tunnel: w207 -> [_ w217]
          frame False {
          }
          frame True {
            n127 = Tick Count (ms)() -> (millisecond timer value=w222:u32)
            n128 = Subtract(x=w222, y=w216) -> (x-y=w221:u32)
            n129 = Equal To 0?(x=w216) -> (x = 0?=w215:bool)
            n130 = Greater Or Equal?(x=w221, y=w217) -> (x >= y?=w219:bool)
            n131 = Select(t=FALSE, s=w215, f=w219) -> ()  [unwired: 1 out]
            n132 = Select(t=w222, s=w215, f=w216) -> (s? t:f=w220:u32)
          }
        }
      }
      frame True {
        n133 = To Double Precision Float(number=w229) -> (double precision float=w228:dbl)
        n134 = Divide(x=w228, y=1000.0) -> (x/y=w225:dbl)
        n135 = call "Get elaphsd time for aiming.vi"("Error in"=w234, "Reset"=w232, "Target time"=w225) -> ("Errorout"=w233:errorcluster, "Elaphshed time"=w226:bool, "Elaphsed time"=→"Elaphsed time":dbl)  [unwired: 6 in]
        n136 = And(x=w230, y=w226) -> (x .and. y?=w231:bool)
      }
    }
    "millisecond timer value" <- w168
    n137 = Compound Arithmetic op=OR(w162, "stop", w154, w151) -> (w180:bool)
  }
  "Camera Refnum in 2" <- w41
  n138 = call "IMAQ Dispose"("Image"=w50, "error in (no error)"=w59) -> ("error out"=w61:errorcluster)  [unwired: 1 in, 3 out]
  n139 = call <vilib>:"IVA Clear Coordsys Errors.vi"("error in (no error)"=w61) -> ("error out"=w60:errorcluster)  [unwired: 10 in]
  n140 = case shown="True" "Check path or camera" {
    tunnel: w60 -> [w430 w433]
    tunnel: [w430 w432] -> w42
    tunnel: w41 -> [_ w431]
    frame False {
    }
    frame True {
      n141 = call <vilib>:"IMAQdx Close Camera.vi"("error in"=w433, "Session In"=w431) -> ("error out"=w432:errorcluster)  [unwired: 9 out]
    }
  }
  n142 = call "IMAQ Dispose"("error in (no error)"=w42) -> ("error out"=w62:errorcluster)  [unwired: 5 in]
  n143 = call <vilib>:"General Error Handler.vi"("error in (no error)"=w62) -> ("error out"=w55:errorcluster)  [unwired: 2 in, 12 out]
  n144 = case shown="False" "Check path or camera" {
    tunnel: w10 -> [_ w435]
    tunnel: [w434 w435] -> w9
    tunnel: "Image" -> [w434 _]
    frame False {
    }
    frame True {
    }
  }
  "Image 2" <- w9
  n145 = property on="Cross Hair Coordinates" class="Clust (strict)"(error in=w55) -> (error out=w19:errorcluster, "Value"=w18:cluster{"X":i32, "Y":i32})  [unwired: 1 in, 1 out]
  n146 = property on="Cross Hair Coordinates 2" class="Clust (strict)"(error in=w19) -> (error out=→"error out 3":errorcluster, "Value"=w15:cluster{"X":i32, "Y":i32})  [unwired: 1 in, 1 out]
  n147 = Unbundle By Name(w18) -> ("X"=w17:i32, "Y"=w16:i32)
  n148 = Unbundle By Name(w15) -> ("X"=w14:i32, "Y"=w13:i32)
  n149 = Bundle By Name(cluster=T2 {"Result"=TRUE, "Exp value X"=0, "Exp value Y"=0, "Act value X "=0, "Act value Y "=0, "Name"=""} ("Cluster"), "Exp value X"=w17, "Exp value Y"=w16, "Act value X"=w14, "Act value Y"=w13, "Result"=w35, "Name"=w20) -> (→"Aiming Result":T2)
